vi "g_Testindicator.vi"() -> ()   [LabVIEW 2014]
panel:
  out "Testindicator":dbl
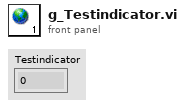
[diagram p1: front panel]
diagram:
